vi "intArrayMaxMin.vi"(8 "Error in (no error)":errorcluster, 11 "Uint array in":refnum<class "IntClass.lvclass">[](array[class])) -> (0 "Error out":errorcluster, 1 "Timing":u32, 2 "Min":refnum<class "IntClass.lvclass">, 3 "Max":refnum<class "IntClass.lvclass">, 4 "Index min":i32, 5 "Index max":i32)   [LabVIEW 2011, in "IntClass.lvclass"]
uses:
  IntClass.lvclass
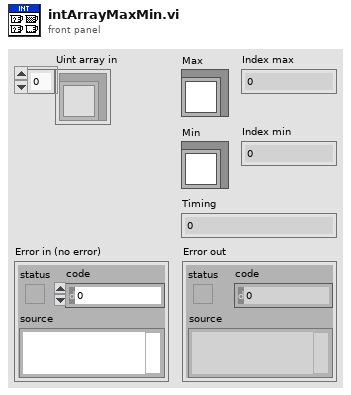
[diagram p1: front panel]
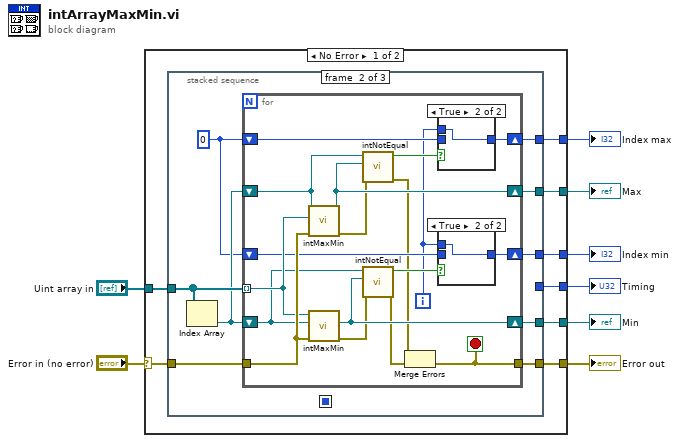
[diagram p0: block diagram]
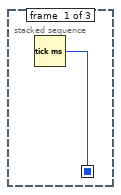
[diagram p2: hidden frame]
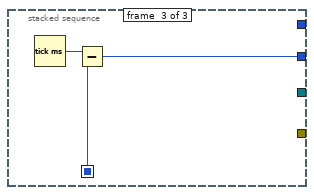
[diagram p5: hidden frame]
diagram:
  n1 = case shown="No Error" "Error in (no error)" {
    selector: "Error in (no error)" -> [w15 w52]
    tunnel: [w14 w52] -> w7
    tunnel: "Uint array in" -> [w16 _]
    tunnel: [w13 _] -> w5
    tunnel: [w12 _] -> w4
    tunnel: [w11 _] -> w3
    tunnel: [w10 _] -> w2
    tunnel: [w9 _] -> w1
    frame No Error {
      n2 = stacked-sequence {
        seq-local: [w17 _ _] -> [_ _ w50]
        tunnel: w16 -> [_ w26 _]
        tunnel: w15 -> [_ w25 _]
        tunnel: [_ w24 _] -> w14
        tunnel: [_ w21 _] -> w13
        tunnel: [_ w20 _] -> w12
        tunnel: [_ w19 _] -> w11
        tunnel: [_ w18 _] -> w10
        tunnel: [_ _ w49] -> w9
        frame #0 {
          n3 = Tick Count (ms)() -> (millisecond timer value=w17:u32)
        }
        frame #1 {
          w22 = 0
          n4 = Index Array(array=w26) -> (element=w23:refnum<class "IntClass.lvclass">)  [unwired: 1 in]
          n5 = for {
            shift-right: [w36] -> w21
            shift-left: w23 -> [w37]
            tunnel: w26 -> [w43] mode=indexing
            shift-right: [w38] -> w20
            shift-left: w23 -> [w39]
            tunnel: w25 -> [w44]
            tunnel: [w27] -> w24
            shift-right: [w40] -> w19
            shift-left: w22 -> [w41]
            shift-right: [w31] -> w18
            shift-left: w22 -> [w32]
            i -> [w30]
            stop <- w27 stop-if-true
            n6 = call "intMaxMin.vi"("Error in (no error)"=w44, "Int2 in"=w43, "Int1 in"=w37) -> ("Error out"=w35:errorcluster, "Max"=w36:refnum<class "IntClass.lvclass">)  [unwired: 5 in, 2 out]
            n7 = call "intMaxMin.vi"("Error in (no error)"=w44, "Int2 in"=w39, "Int1 in"=w43) -> ("Error out"=w34:errorcluster, "Min"=w38:refnum<class "IntClass.lvclass">)  [unwired: 5 in, 2 out]
            n8 = call "intNotEqual.vi"("Error in (no error)"=w35, "Int2 in"=w36, "Int1 in"=w37) -> ("Error out"=w29:errorcluster, "Int1 != Int2?"=w42:bool)  [unwired: 6 in, 1 out]
            n9 = call "intNotEqual.vi"("Error in (no error)"=w34, "Int2 in"=w38, "Int1 in"=w39) -> ("Error out"=w28:errorcluster, "Int1 != Int2?"=w33:bool)  [unwired: 6 in, 1 out]
            n10 = Merge Errors(w29, w28) -> (w27:errorcluster)
            n11 = case shown="True" w42 {
              tunnel: w41 -> [w47 _]
              tunnel: [w47 w48] -> w40
              tunnel: w30 -> [_ w48]
              frame False {
              }
              frame True {
              }
            }
            n12 = case shown="True" w33 {
              tunnel: w32 -> [w45 _]
              tunnel: [w45 w46] -> w31
              tunnel: w30 -> [_ w46]
              frame False {
              }
              frame True {
              }
            }
          }
        }
        frame #2 {
          n13 = Tick Count (ms)() -> (millisecond timer value=w51:u32)
          n14 = Subtract(x=w51, y=w50) -> (x-y=w49:u32)
        }
      }
    }
    frame Error {
    }
  }
  "Error out" <- w7
  "Max" <- w5
  "Timing" <- w1
  "Min" <- w4
  "Index max" <- w3
  "Index min" <- w2
